vi "Process.vi"(8 "error in":errorcluster, 11 "Plugin in":refnum<class "FFT.lvclass">) -> (0 "error out":errorcluster, 3 "Plugin out":refnum<class "FFT.lvclass">)   [LabVIEW 2024, in "FFT.lvlib" / "FFT.lvclass"]
uses:
  FFT.lvclass
  C:/Program Files/National Instruments/LabVIEW 2024/vi.lib/FlexLogger/SDK/PluginSDK.lvlibp/PEFClasses/SDK/Plugin/Plugin.lvclass
  FFT Buffer Manager Function.ctl
  <vilib>/Analysis/2dsp.llb/Power Spectrum (DBL).vi
  <vilib>/FlexLogger/SDK/PluginSDK.lvlibp/PEFClasses/SDK/Producer Channel/Producer Channel.lvclass
  C:/Program Files/National Instruments/LabVIEW 2024/vi.lib/FlexLogger/SDK/PluginSDK.lvlibp/PEFClasses/SDK/Channel/Channel.lvclass
  FFT Globals.vi
  <vilib>/FlexLogger/SDK/PluginSDK.lvlibp/PEFClasses/SDK/Channel/ParameterAccess/Read I32.vi
  <vilib>/FlexLogger/SDK/PluginSDK.lvlibp/PEFClasses/SDK/Channel/ParameterAccess/Read Boolean.vi
  <vilib>/FlexLogger/SDK/PluginSDK.lvlibp/PEFClasses/SDK/Plugin/DataHelpers/Write 2D DBL (NChan NSamples).vi
  <vilib>/FlexLogger/SDK/PluginSDK.lvlibp/PEFClasses/SDK/Plugin/Plugin.lvclass
  <vilib>/Analysis/NI_AALPro.lvlib
  <vilib>/FlexLogger/SDK/PluginSDK.lvlibp/PEFClasses/SDK/Channel/Channel.lvclass
  C:/Program Files/National Instruments/LabVIEW 2024/vi.lib/FlexLogger/SDK/PluginSDK.lvlibp/PEFClasses/SDK/Processing Element/Processing Element.lvclass
  C:/Users/Administrator/Documents/LabVIEW Projects/FlexLogger IO Plug-ins/FFT/FFT.lvclass
  C:/Program Files/National Instruments/LabVIEW 2024/vi.lib/FlexLogger/SDK/PluginSDK.lvlibp/PEFClasses/SDK/Producer Channel/Producer Channel.lvclass
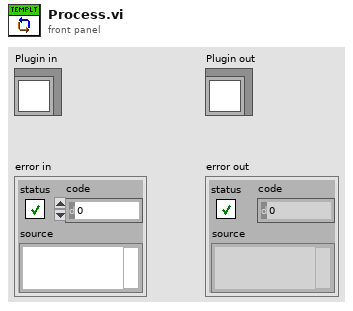
[diagram p1: front panel]
types:
  T1 = typedef "FFT.lvlib/FFT.lvclass/FFT Buffer Manager Function.ctl" = enum16{"Get Data", "Buffer Data", "Reset Data"}
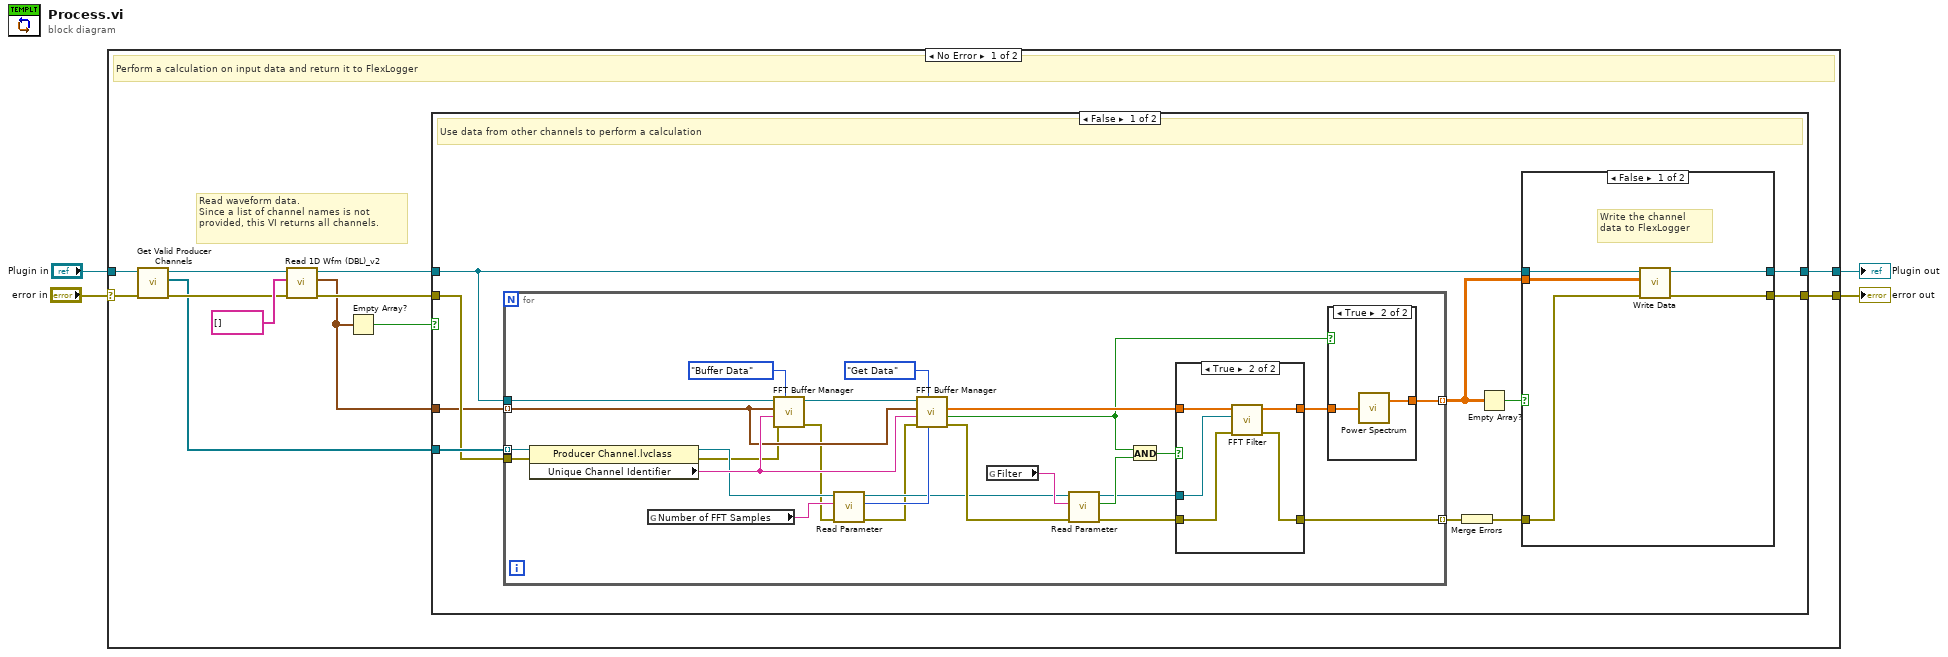
[diagram p0: block diagram]
diagram:
  n1 = case shown="No Error" "error in" {
    selector: "error in" -> [w9 w71]
    tunnel: [w15 w72] -> w1
    tunnel: "Plugin in" -> [w11 w72]
    tunnel: [w16 w71] -> w2
    frame No Error {
      # "Read waveform data.\nSince a list of channel names is not provided, this VI returns all channels."
      # "Perform a calculation on input data and return it to FlexLogger"
      n2 = call <vilib>:"Get Valid Producer Channels.vi"("error in (no error)"=w9, "Plugin in"=w11) -> ("error out"=w8:errorcluster, "Channels"=w7:refnum<class "Producer Channel.lvclass">[], "Plugin out"=w10:refnum<class "FFT.lvclass">)  [unwired: 7 in]
      n3 = call <vilib>:"Read 1D Wfm (DBL)_v2.vi"("error in (no error)"=w8, "Unique Identifers (empty = all)"=string[] [] ("Unique Channel Identifers (empty = all)"), "Plugin in"=w10) -> ("error out"=w14:errorcluster, "Data"=w5:waveform(dbl)[], "Plugin out"=w12:refnum<class "FFT.lvclass">)  [unwired: 5 in, 1 out]
      n4 = Empty Array?(array=w5) -> (empty?=w6:bool)
      n5 = case shown="False" w6 {
        tunnel: [w26 w69] -> w16
        tunnel: [w25 w70] -> w15
        tunnel: w12 -> [w24 w70]
        tunnel: w14 -> [w22 w69]
        tunnel: w7 -> [w23 _]
        tunnel: w5 -> [w21 _]
        frame False {
          # "Use data from other channels to perform a calculation"
          n6 = for {
            tunnel: w24 -> [w38]
            tunnel: [w56] -> w20 mode=indexing
            tunnel: w23 -> [w43] mode=indexing
            tunnel: w22 -> [w36]
            tunnel: w21 -> [w37] mode=indexing
            tunnel: [w39] -> w18 mode=indexing
            n7 = property class="Producer Channel.lvclass"(reference=w43, error in=w36) -> (reference out=w42:refnum<class "Producer Channel.lvclass">, error out=w35:errorcluster, "Unique Channel Identifier"=w44:string)
            n8 = global read "FFT Globals.vi" "Number of FFT Samples"() -> (w54:string)
            n9 = call "FFT Buffer Manager.vi"("Function"=FFT_Buffer_Manager_Function."Buffer Data", "error in"=w35, "Unique Channel Identifier"=w44, "Waveform"=w37, "Plugin in"=w38) -> ("error out"=w34:errorcluster, "Plugin out"=w58:refnum<class "FFT.lvclass">)  [unwired: 3 in, 2 out]
            n10 = call-poly <vilib>:"Read Parameter.vi"("error in (no error)"=w34, "Name"=w54, "Channel in"=w42) -> ("error out"=w40:errorcluster, "Value"=w52:i32, "Channel out"=w41:refnum<class "Producer Channel.lvclass">)  [unwired: 5 in, 1 out]
            n11 = call "FFT Buffer Manager.vi"("FFT Samples"=w52, "Function"=FFT_Buffer_Manager_Function."Get Data", "error in"=w40, "Unique Channel Identifier"=w44, "Waveform"=w37, "Plugin in"=w58) -> ("error out"=w53:errorcluster, "Data Valid"=w49:bool, "Data"=w51:dbl[])  [unwired: 2 in, 1 out]
            n12 = global read "FFT Globals.vi" "Filter"() -> (w55:string)
            n13 = call-poly <vilib>:"Read Parameter.vi"("error in (no error)"=w53, "Name"=w55, "Channel in"=w41) -> ("error out"=w45:errorcluster, "Value"=w48:bool, "Channel out"=w46:refnum<class "Producer Channel.lvclass">)  [unwired: 5 in, 1 out]
            n14 = And(x=w49, y=w48) -> (x .and. y?=w47:bool)
            n15 = case shown="True" w47 {
              tunnel: w51 -> [w61 w66]
              tunnel: [w61 w64] -> w50
              tunnel: w46 -> [_ w63]
              tunnel: w45 -> [w60 w65]
              tunnel: [w60 w62] -> w39
              frame False {
              }
              frame True {
                n16 = call "FFT Filter.vi"("error in"=w65, "Channel in"=w63, "Data in"=w66) -> ("error out"=w62:errorcluster, "Data out"=w64:dbl[])  [unwired: 7 in]
              }
            }
            n17 = case shown="True" w49 {
              tunnel: w50 -> [_ w68]
              tunnel: [_ w67] -> w56
              frame False {
              }
              frame True {
                n18 = call-poly <vilib>:"Power Spectrum.vi"("X"=w68) -> ("Power Spectrum"=w67:dbl[])  [unwired: 1 out]
              }
            }
          }
          n19 = Merge Errors(w18) -> (w17:errorcluster)
          n20 = Empty Array?(array=w20) -> (empty?=w19:bool)
          n21 = case shown="False" w19 {
            tunnel: [w31 w32] -> w26
            tunnel: [w30 w33] -> w25
            tunnel: w24 -> [w29 w33]
            tunnel: w20 -> [w28 _]
            tunnel: w17 -> [w27 w32]
            frame False {
              # "Write the channel data to FlexLogger"
              n22 = call-poly <vilib>:"Write Data.vi"("error in (no error)"=w27, "Data"=w28, "Plugin in"=w29) -> ("error out"=w31:errorcluster, "Plugin out"=w30:refnum<class "FFT.lvclass">)  [unwired: 7 in]
            }
            frame True {
            }
          }
        }
        frame True {
          # "No channels sending data to the plugin"
        }
      }
    }
    frame Error {
    }
  }
  "error out" <- w2
  "Plugin out" <- w1
